vi "make_axes_main.vi"(5 "Value Pair Properties":T5={"X Value Pairs"={"Data Array"=[], "Show ticks"=TRUE, "Show grid lines"=TRUE, "Labels"=enum."Name"}, "Y Value Pairs"={"Data Array"=[], "Show ticks"=TRUE, "Show grid lines"=TRUE, "Labels"=enum."Value"}, "Z Value Pairs"={"Data Array"=[], "Show ticks"=TRUE, "Show grid lines"=TRUE, "Labels"=enum."Value"}}, 6 "Format strings":T2, 7 "Axes Properties":T7={"Grid  Properties"={"Grid Visible"={"Draw X-grid"=FALSE, "Draw Y-grid"=FALSE, "Draw Z-grid"=FALSE}, "Grid Color"={"Color X"=0, "Color Y"=0, "Color Z"=0}}, "Ticks Properties"={"Minor Count"={"X"=0, "Y"=0, "Z"=0}, "Major Count"={"X"=0, "Y"=0, "Z"=0}, "Major Ticks Visible"={"X"=FALSE, "Y"=FALSE, "Z"=FALSE}, "Minor Ticks Visible"={"X"=FALSE, "Y"=FALSE, "Z"=FALSE}, "Tick Color"={"Color X"=0, "Color Y"=0, "Color Z"=0}}, "from/to cluster"={"X"={"Min"=0.0, "Max"=0.0}, "Y"={"Min"=0.0, "Max"=0.0}, "Z"={"Min"=0.0, "Max"=0.0}, "Amplitude"={"Min"=0.0, "Max"=0.0}}, "Caption Properties"={"Show Captions"={"Show X Caption"=FALSE, "Show Z Caption"=TRUE, "Show Y Caption"=TRUE, "Show Opposite X Caption"=FALSE, "Show Opposite Y Caption"=TRUE, "Show Opposite Z Caption"=TRUE}, "Captions"={"Caption X"="", "Caption Y"="", "Caption Z"=""}, "Caption Color"={"Color X"=0, "Color Y"=0, "Color Z"=0}, "Caption Font Size"={"Font Size X"=12, "Font Size Y"=12, "Font Size Z"=12}}, "Labels Properties"={"Label Visible"={"Show X Labels"=FALSE, "Show Y Labels"=FALSE, "Show Z Labels"=FALSE, "Show Opposite X Labels"=FALSE, "Show Opposite Y Labels"=FALSE, "Show Opposite Z Labels"=FALSE}, "Label Color"={"Color X"=0, "Color Y"=0, "Color Z"=0}, "Label Font Size"={"Font Size X"=0, "Font Size Y"=0, "Font Size Z"=0}}, "Auto Range On"={"X"=TRUE, "Y"=TRUE, "Z"=TRUE}}, 8 "length":sgl, 9 "Range Min/Max":T3={"X"={"Min"=inf, "Max"=-inf}, "Y"={"Min"=inf, "Max"=-inf}, "Z"={"Min"=inf, "Max"=-inf}, "Amplitude"={"Min"=0.0, "Max"=0.0}}, 10 "Graph Properties":T1, 11 "Grid Scene Object In":refnum<vi>) -> (3 "Grid Scene Object Out":refnum<vi>)   [LabVIEW 2020, in "3DPC_SurfacePlot.xctl"]
uses:
  <vilib>/Native 3D Graph/xcontrol/3DPC_SurfacePlot.xctl
  <vilib>/Native 3D Graph/typedefs/prop_axes_all.ctl
  <vilib>/Native 3D Graph/typedefs/prop_axes_grid.ctl
  <vilib>/Native 3D Graph/typedefs/prop_axes_ticks.ctl
  <vilib>/Native 3D Graph/typedefs/range_cluster.ctl
  <vilib>/Native 3D Graph/typedefs/min_max.ctl
  <vilib>/Native 3D Graph/typedefs/prop_axes_captions.ctl
  <vilib>/Native 3D Graph/typedefs/prop_axes_labels.ctl
  <vilib>/Native 3D Graph/typedefs/prop_axes_autorange.ctl
  <vilib>/Native 3D Graph/typedefs/prop_value_pair_all.ctl
  <vilib>/Native 3D Graph/typedefs/prop_value_pair_1d.ctl
  <vilib>/Native 3D Graph/typedefs/prop_format.ctl
  <vilib>/Native 3D Graph/typedefs/prop_graph.ctl
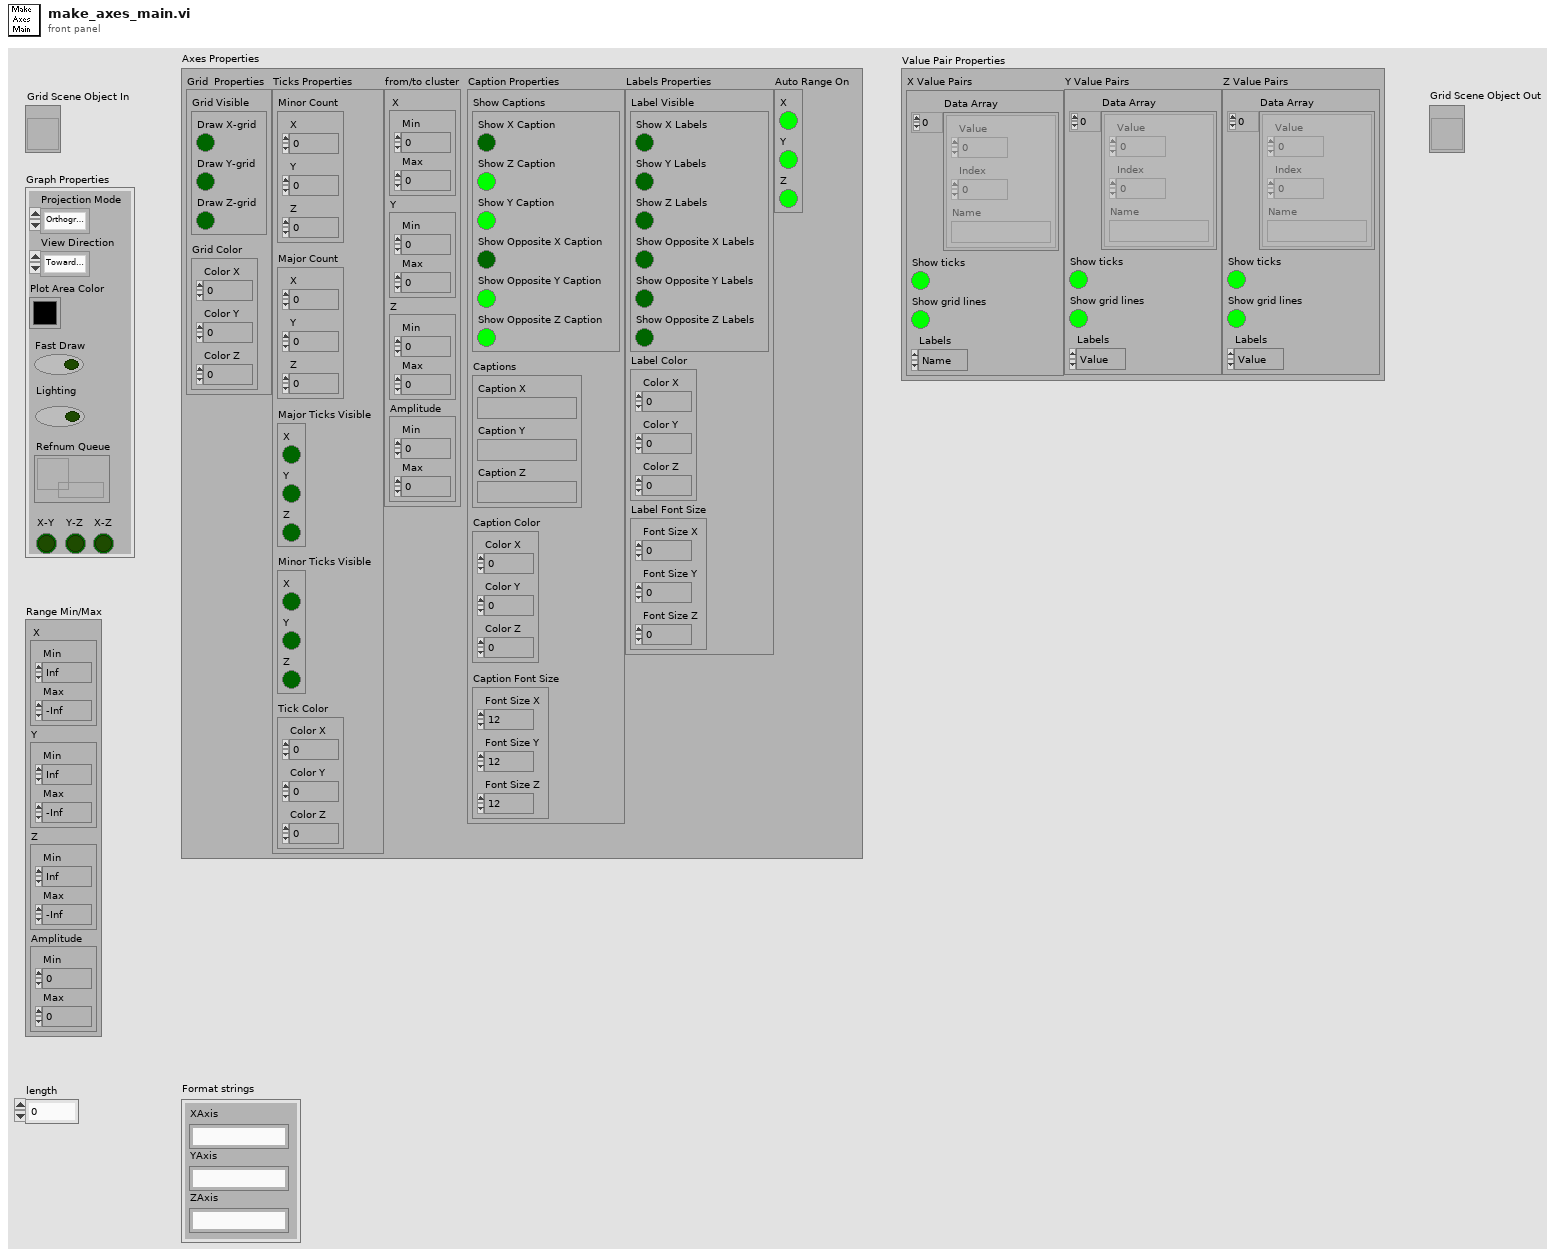
[diagram p1: front panel]
types:
  T1 = typedef "3DPC_SurfacePlot.xctl/prop_graph.ctl" = cluster{"Projection Mode":enum16{"Orthographic", "Perspective"}, "View Direction":enum32{"Towards X-Y Plane", "Towards Y-Z Plane", "Towards X-Z Plane", "User Define"}, "Plot Area Color":u32, "Fast Draw":bool, "X-Y":bool, "Y-Z":bool, "X-Z":bool, "Lighting":bool, "Refnum Queue":refnum<queue>}
  T2 = typedef "3DPC_SurfacePlot.xctl/prop_format.ctl" = cluster{"XAxis":string, "YAxis":string, "ZAxis":string}
  T3 = typedef "3DPC_SurfacePlot.xctl/range_cluster.ctl" = cluster{"X":T4, "Y":T4, "Z":T4, "Amplitude":T4}
  T4 = typedef "3DPC_SurfacePlot.xctl/min_max.ctl" = cluster{"Min":sgl, "Max":sgl}
  T5 = typedef "3DPC_SurfacePlot.xctl/prop_value_pair_all.ctl" = cluster{"X Value Pairs":cluster{"Data Array":cluster{"Value":sgl, "Index":i32, "Name":string}[], "Show ticks":bool, "Show grid lines":bool, "Labels":enum16{"Value", "None", "Name"}}, "Y Value Pairs":T6, "Z Value Pairs":T6}
  T6 = typedef "3DPC_SurfacePlot.xctl/prop_value_pair_1d.ctl" = cluster{"Data Array":cluster{"Value":sgl, "Index":i32, "Name":string}[], "Show ticks":bool, "Show grid lines":bool, "Labels":enum16{"Value", "None", "Name"}}
  T7 = typedef "3DPC_SurfacePlot.xctl/prop_axes_all.ctl" = cluster{"Grid  Properties":T8, "Ticks Properties":T9, "from/to cluster":T3, "Caption Properties":T10, "Labels Properties":T11, "Auto Range On":T12}
  T8 = typedef "3DPC_SurfacePlot.xctl/prop_axes_grid.ctl" = cluster{"Grid Visible":cluster{"Draw X-grid":bool, "Draw Y-grid":bool, "Draw Z-grid":bool}, "Grid Color":cluster{"Color X":u32, "Color Y":u32, "Color Z":u32}}
  T9 = typedef "3DPC_SurfacePlot.xctl/prop_axes_ticks.ctl" = cluster{"Minor Count":cluster{"X":i32, "Y":i32, "Z":i32}, "Major Count":cluster{"X":i32, "Y":i32, "Z":i32}, "Major Ticks Visible":cluster{"X":bool, "Y":bool, "Z":bool}, "Minor Ticks Visible":cluster{"X":bool, "Y":bool, "Z":bool}, "Tick Color":cluster{"Color X":u32, "Color Y":u32, "Color Z":u32}}
  T10 = typedef "3DPC_SurfacePlot.xctl/prop_axes_captions.ctl" = cluster{"Show Captions":cluster{"Show X Caption":bool, "Show Z Caption":bool, "Show Y Caption":bool, "Show Opposite X Caption":bool, "Show Opposite Y Caption":bool, "Show Opposite Z Caption":bool}, "Captions":cluster{"Caption X":string, "Caption Y":string, "Caption Z":string}, "Caption Color":cluster{"Color X":u32, "Color Y":u32, "Color Z":u32}, "Caption Font Size":cluster{"Font Size X":i16, "Font Size Y":i16, "Font Size Z":i16}}
  T11 = typedef "3DPC_SurfacePlot.xctl/prop_axes_labels.ctl" = cluster{"Label Visible":cluster{"Show X Labels":bool, "Show Y Labels":bool, "Show Z Labels":bool, "Show Opposite X Labels":bool, "Show Opposite Y Labels":bool, "Show Opposite Z Labels":bool}, "Label Color":cluster{"Color X":u32, "Color Y":u32, "Color Z":u32}, "Label Font Size":cluster{"Font Size X":i16, "Font Size Y":i16, "Font Size Z":i16}}
  T12 = typedef "3DPC_SurfacePlot.xctl/prop_axes_autorange.ctl" = cluster{"X":bool, "Y":bool, "Z":bool}
  T13 = enum32{"Towards X-Y Plane", "Towards Y-Z Plane", "Towards X-Z Plane", "User Define"}
  T14 = typedef "3DPC_SurfacePlot.xctl/prop_axes_merged_array_etc.ctl" = cluster{"X Merged Array":T15, "Y Merged Array":T15, "Z Merged Array":T15, "Range Min/Max":T3}
  T15 = typedef "3DPC_SurfacePlot.xctl/prop_axes_merged_array.ctl" = cluster{"Show Tick":bool, "Show Line":bool, "Interval":sgl, "Name":string}[]
  T16 = cluster{"X Label Width":dbl, "Y Label Width":dbl, "Z Label Width":dbl, "X Label Width Opposite":dbl, "Y Label Width Opposite":dbl, "Z Label Width Opposite":dbl}
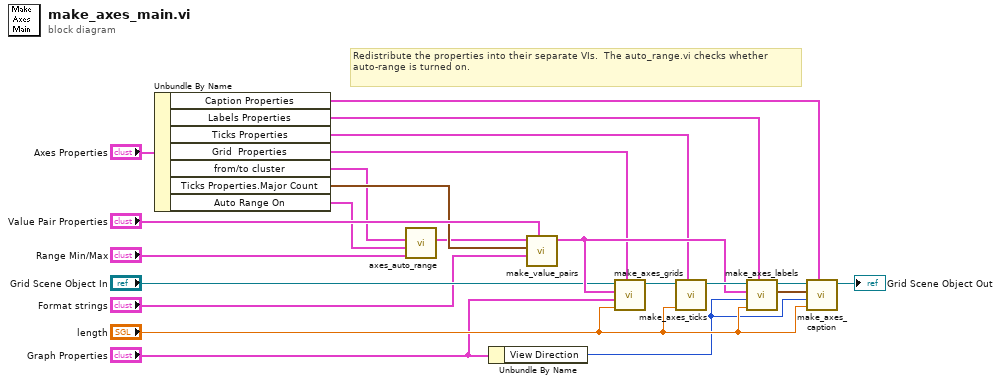
[diagram p0: block diagram]
diagram:
  # "Redistribute the properties into their separate VIs.  The auto_range.vi checks whether auto-range is turned on."
  n1 = Unbundle By Name("Axes Properties") -> ("Caption Properties"=w9:T10, "Labels Properties"=w8:T11, "Ticks Properties"=w11:T9, "Grid  Properties"=w12:T8, "from/to cluster"=w6:T3, "Ticks Properties.Major Count"=w13:cluster{"X":i32, "Y":i32, "Z":i32}, "Auto Range On"=w5:T12)
  n2 = call <vilib>:"axes_auto_range.vi"("Acutal Range"="Range Min/Max", "Auto Range On"=w5, "Set Range To"=w6) -> ("Range Min/Max"=w4:T3)  [unwired: 8 out]
  n3 = Unbundle By Name("Graph Properties") -> ("View Direction"=w1:T13)
  n4 = call <vilib>:"make_value_pairs.vi"("Value Pair Properties"="Value Pair Properties", "Format strings"="Format strings", "Ticks Properties.Major Count"=w13, "Range Min/Max"=w4) -> ("Axis output cluster"=w16:T14)  [unwired: 1 in, 6 out]
  n5 = call <vilib>:"make_axes_grids.vi"("Grid  Properties"=w12, "length"="length", "Graph Properties"="Graph Properties", "Axis output cluster"=w16, "Scene Object In"="Grid Scene Object In") -> ("Scene Object Out"=w22:refnum<vi>)  [unwired: 6 out]
  n6 = call <vilib>:"make_axes_ticks.vi"("Ticks Properties"=w11, "length"="length", "Scene Object In"=w22) -> ("Scene Object Out"=w21:refnum<vi>)  [unwired: 1 in, 7 out]
  n7 = call <vilib>:"make_axes_labels.vi"("Labels Properties"=w8, "length"="length", "View Direction"=w1, "Axis output cluster"=w16, "Scene Object In"=w21) -> ("Label Width"=w17:T16, "Scene Object Out"=w18:refnum<vi>)  [unwired: 5 out]
  n8 = call <vilib>:"make_axes_caption.vi"("Caption Properties"=w9, "Length"="length", "View Direction"=w1, "Label Width"=w17, "Scene Object In"=w18) -> ("Scene Object Out"=→"Grid Scene Object Out":refnum<vi>)  [unwired: 6 out]
